vi "Avg_MaxV2.vi"(10 "# of Max":i32, 11 "Array":dbl[](array[numeric])) -> (3 "Avg Max":dbl)   [LabVIEW 2014]
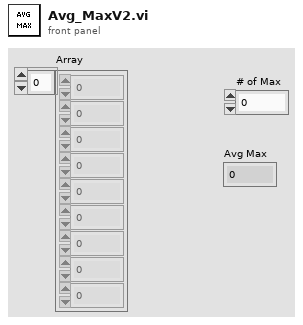
[diagram p1: front panel]
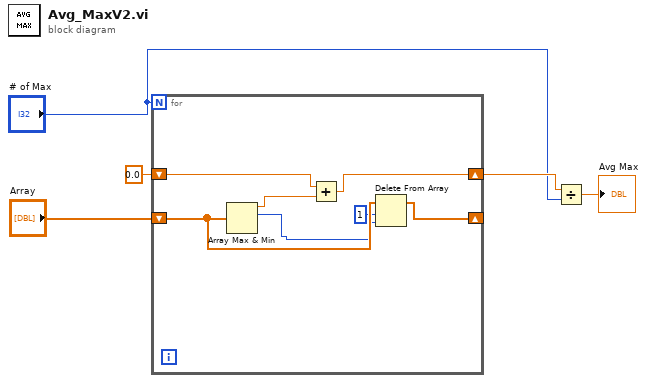
[diagram p0: block diagram]
diagram:
  n1 = for {
    N: "# of Max" -> [_]
    shift-right: [w8] -> _
    shift-left: "Array" -> [w12]
    shift-right: [w10] -> w3
    shift-left: 0.0 -> [w9]
    n2 = Array Max & Min(array=w12) -> (max value=w7:dbl, max index (indices)=w6:i32)  [unwired: 2 out]
    n3 = Add(x=w9, y=w7) -> (x+y=w10:dbl)
    n4 = Delete From Array(array=w12, length=1, index=w6) -> (array with subset deleted=w8:dbl[])  [unwired: 1 out]
  }
  n5 = Divide(x=w3, y="# of Max") -> (x/y=→"Avg Max":dbl)
